vi "Trigger and Confirm.vi"(5 "Timestamp Channel (Confirm)":string, 6 "Timeout (s)":dbl=20.0 format="%#_13g", 7 "Trigger Channel":string, 8 "error in (no error)":errorcluster, 10 "Number of Triggers":i32=1, 11 "WorkspaceManager in":T1) -> (0 "error out":errorcluster, 3 "WorkspaceManager out":T1)   [LabVIEW 2018, in "Instrument Addon Common System Tests.lvclass"]
uses:
  Instrument Addon Common System Tests.lvclass
  <vilib>/NI Veristand/Execution/Workspace/WorkspaceAPI.ctl
  NationalInstruments.VeriStand.ClientAPI
  <vilib>/NI Veristand/Execution/Workspace/NI VeriStand - Get Single Channel Value.vi
  <vilib>/NI Veristand/Execution/Workspace/NI VeriStand - Set Single Channel Value.vi
  <vilib>/NI Veristand/Execution/Workspace/NI_VS Workspace ExecutionAPI.lvlib
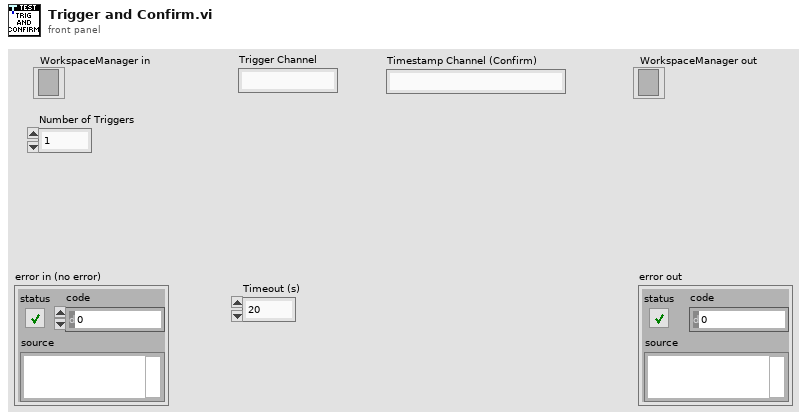
[diagram p1: front panel]
types:
  T1 = typedef "NI_VS Workspace ExecutionAPI.lvlib/WorkspaceAPI.ctl" = refnum<k24>
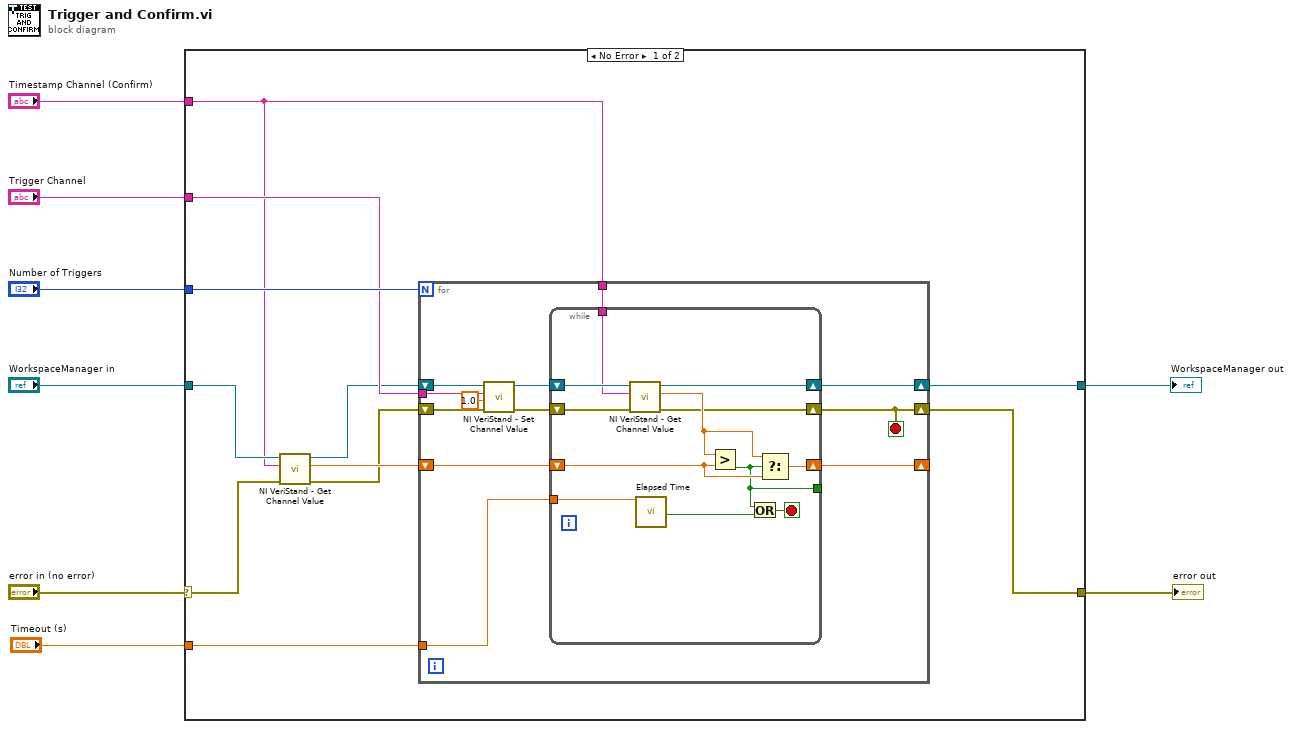
[diagram p0: block diagram]
diagram:
  n1 = case shown="No Error" "error in (no error)" {
    selector: "error in (no error)" -> [w10 w44]
    tunnel: "Number of Triggers" -> [w19 _]
    tunnel: [w18 w44] -> w7
    tunnel: "Trigger Channel" -> [w17 _]
    tunnel: "WorkspaceManager in" -> [w14 w45]
    tunnel: "Timestamp Channel (Confirm)" -> [w12 _]
    tunnel: [w11 w45] -> w3
    tunnel: "Timeout (s)" -> [w9 _]
    frame No Error {
      n2 = call-poly <vilib>:"NI VeriStand - Get Channel Value.vi"("error in (no error)"=w10, "Channel"=w12, "WorkspaceManager in"=w14) -> ("error out"=w15:errorcluster, "Value"=w16:dbl, "WorkspaceManager out"=w13:T1)  [unwired: 6 in]
      n3 = for {
        N: w19 -> [_]
        tunnel: w17 -> [w31]
        shift-right: [w22] -> w18
        shift-left: w15 -> [w26]
        shift-right: [w24] -> w11
        shift-left: w13 -> [w29]
        tunnel: w12 -> [w25]
        shift-right: [w23] -> _
        shift-left: w16 -> [w28]
        tunnel: w9 -> [w20]
        stop <- w22 stop-if-true
        n4 = call-poly <vilib>:"NI VeriStand - Set Channel Value.vi"("error in (no error)"=w26, "Value"=1.0, "Channel"=w31, "WorkspaceManager in"=w29) -> ("error out"=w27:errorcluster, "WorkspaceManager out"=w30:T1)  [unwired: 6 in]
        n5 = while {
          shift-right: [w41] -> w24
          shift-left: w30 -> [w43]
          shift-right: [w33] -> w22
          shift-left: w27 -> [w42]
          shift-right: [w40] -> w23
          shift-left: w28 -> [w35]
          tunnel: [w34] -> _
          tunnel: w25 -> [w37]
          tunnel: w20 -> [w32]
          stop <- w38 stop-if-true
          n6 = call-poly <vilib>:"NI VeriStand - Get Channel Value.vi"("error in (no error)"=w42, "Channel"=w37, "WorkspaceManager in"=w43) -> ("error out"=w33:errorcluster, "Value"=w36:dbl, "WorkspaceManager out"=w41:T1)  [unwired: 6 in]
          n7 = call "Elapsed Time"("Time Target (s)"=w32) -> ("Time has Elapsed"=w39:bool)  [unwired: 11 in, 7 out]
          n8 = Greater?(x=w36, y=w35) -> (0:w34:bool)
          n9 = Or(x=w34, y=w39) -> (x .or. y?=w38:bool)
          n10 = Select(t=w36, s=w34, f=w35) -> (s? t:f=w40:dbl)
        }
      }
    }
    frame Error {
    }
  }
  "error out" <- w7
  "WorkspaceManager out" <- w3
